vi "烟雾监测界面.vi"() -> ()   [LabVIEW 2016, in "环境动力监测库.lvlib"]
panel:
  out "x+1":u32
  in  "解除告警":bool
  out "告警内容":string
  out "X5-烟雾检测_YW":bool caption="状态"
  # "烟雾监测"
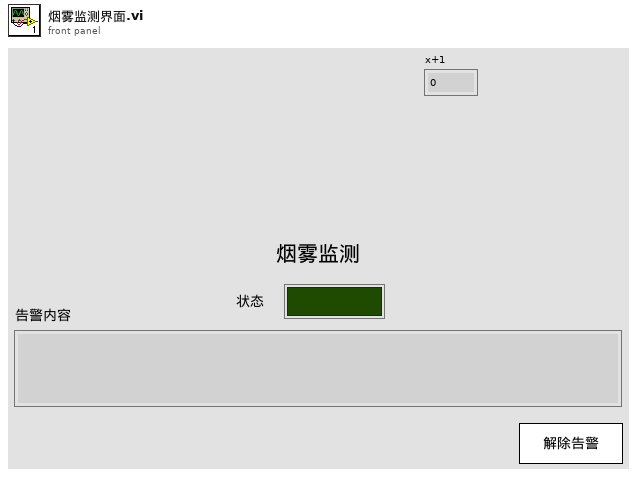
[diagram p1: front panel]
types:
  T1 = cluster{"漏水监测配置":cluster{"监测项描述:输出":string, "端口:":enum16{"AI0", "AI1", "AI2", "AI3", "AI4", "DI0", "DI1", "DI2", "DI3", "DI4", "DO0", "DO1", "DO2", "DO3", "DO4", "X0", "X1", "X2", "X3", "X4", "X5", "X6", "X7", "X8", "X9", "X10", "X11", "X12", "X13", "X14", "X15", "X16", "X17", "X18", "X19", "X20", "X21", "X22", "X23"}, "告警参数:":enum32{"禁用告警", "闭合告警", "断开告警"}, "传感器型号:":enum16{"PLC", "ZLAN", "ART"}, "声光告警启用":bool}, "门禁开关监测配置":cluster{"监测项描述:输出":string, "端口:":enum16{"AI0", "AI1", "AI2", "AI3", "AI4", "DI0", "DI1", "DI2", "DI3", "DI4", "DO0", "DO1", "DO2", "DO3", "DO4", "X0", "X1", "X2", "X3", "X4", "X5", "X6", "X7", "X8", "X9", "X10", "X11", "X12", "X13", "X14", "X15", "X16", "X17", "X18", "X19", "X20", "X21", "X22", "X23"}, "告警参数:":enum32{"禁用告警", "闭合告警", "断开告警"}, "传感器型号:":enum16{"PLC", "ZLAN", "ART"}, "声光告警启用":bool}, "门禁开关监测配置2":cluster{"监测项描述:输出":string, "端口:":enum16{"AI0", "AI1", "AI2", "AI3", "AI4", "DI0", "DI1", "DI2", "DI3", "DI4", "DO0", "DO1", "DO2", "DO3", "DO4", "X0", "X1", "X2", "X3", "X4", "X5", "X6", "X7", "X8", "X9", "X10", "X11", "X12", "X13", "X14", "X15", "X16", "X17", "X18", "X19", "X20", "X21", "X22", "X23"}, "告警参数:":enum32{"禁用告警", "闭合告警", "断开告警"}, "传感器型号:":enum16{"PLC", "ZLAN", "ART"}, "声光告警启用":bool}, "温湿度监测配置":cluster{"监测项描述:输出":string, "端口:":enum16{"AI0", "AI1", "AI2", "AI3", "AI4", "DI0", "DI1", "DI2", "DI3", "DI4", "DO0", "DO1", "DO2", "DO3", "DO4", "X0", "X1", "X2", "X3", "X4", "X5", "X6", "X7", "X8", "X9", "X10", "X11", "X12", "X13", "X14", "X15", "X16", "X17", "X18", "X19", "X20", "X21", "X22", "X23"}, "告警参数:":enum32{"禁用告警", "闭合告警", "断开告警"}, "传感器型号:":enum16{"PLC", "ZLAN", "ART"}, "声光告警启用":bool}, "烟雾监测配置":cluster{"监测项描述:输出":string, "端口:":enum16{"AI0", "AI1", "AI2", "AI3", "AI4", "DI0", "DI1", "DI2", "DI3", "DI4", "DO0", "DO1", "DO2", "DO3", "DO4", "X0", "X1", "X2", "X3", "X4", "X5", "X6", "X7", "X8", "X9", "X10", "X11", "X12", "X13", "X14", "X15", "X16", "X17", "X18", "X19", "X20", "X21", "X22", "X23"}, "告警参数:":enum32{"禁用告警", "闭合告警", "断开告警"}, "传感器型号:":enum16{"PLC", "ZLAN", "ART"}, "声光告警启用":bool}, "冰箱监测配置":cluster{"监测项描述:输出":string, "端口:":enum16{"AI0", "AI1", "AI2", "AI3", "AI4", "DI0", "DI1", "DI2", "DI3", "DI4", "DO0", "DO1", "DO2", "DO3", "DO4", "X0", "X1", "X2", "X3", "X4", "X5", "X6", "X7", "X8", "X9", "X10", "X11", "X12", "X13", "X14", "X15", "X16", "X17", "X18", "X19", "X20", "X21", "X22", "X23"}, "告警参数:":enum32{"禁用告警", "闭合告警", "断开告警"}, "传感器型号:":enum16{"PLC", "ZLAN", "ART"}, "声光告警启用":bool}, "排气扇监测配置":cluster{"监测项描述:输出":string, "端口:":enum16{"AI0", "AI1", "AI2", "AI3", "AI4", "DI0", "DI1", "DI2", "DI3", "DI4", "DO0", "DO1", "DO2", "DO3", "DO4", "X0", "X1", "X2", "X3", "X4", "X5", "X6", "X7", "X8", "X9", "X10", "X11", "X12", "X13", "X14", "X15", "X16", "X17", "X18", "X19", "X20", "X21", "X22", "X23"}, "告警参数:":enum32{"禁用告警", "闭合告警", "断开告警"}, "传感器型号:":enum16{"PLC", "ZLAN", "ART"}, "声光告警启用":bool}, "红外入侵监测配置":cluster{"监测项描述:输出":string, "端口:":enum16{"AI0", "AI1", "AI2", "AI3", "AI4", "DI0", "DI1", "DI2", "DI3", "DI4", "DO0", "DO1", "DO2", "DO3", "DO4", "X0", "X1", "X2", "X3", "X4", "X5", "X6", "X7", "X8", "X9", "X10", "X11", "X12", "X13", "X14", "X15", "X16", "X17", "X18", "X19", "X20", "X21", "X22", "X23"}, "告警参数:":enum32{"禁用告警", "闭合告警", "断开告警"}, "传感器型号:":enum16{"PLC", "ZLAN", "ART"}, "声光告警启用":bool}, "振动监测配置":cluster{"监测项描述:输出":string, "端口:":enum16{"AI0", "AI1", "AI2", "AI3", "AI4", "DI0", "DI1", "DI2", "DI3", "DI4", "DO0", "DO1", "DO2", "DO3", "DO4", "X0", "X1", "X2", "X3", "X4", "X5", "X6", "X7", "X8", "X9", "X10", "X11", "X12", "X13", "X14", "X15", "X16", "X17", "X18", "X19", "X20", "X21", "X22", "X23"}, "告警参数:":enum32{"禁用告警", "闭合告警", "断开告警"}, "传感器型号:":enum16{"PLC", "ZLAN", "ART"}, "声光告警启用":bool}}
  T2 = cluster{"监测项描述:输出":string, "端口:":enum16{"AI0", "AI1", "AI2", "AI3", "AI4", "DI0", "DI1", "DI2", "DI3", "DI4", "DO0", "DO1", "DO2", "DO3", "DO4", "X0", "X1", "X2", "X3", "X4", "X5", "X6", "X7", "X8", "X9", "X10", "X11", "X12", "X13", "X14", "X15", "X16", "X17", "X18", "X19", "X20", "X21", "X22", "X23"}, "告警参数:":enum32{"禁用告警", "闭合告警", "断开告警"}, "传感器型号:":enum16{"PLC", "ZLAN", "ART"}, "声光告警启用":bool}
  T3 = enum16{"AI0", "AI1", "AI2", "AI3", "AI4", "DI0", "DI1", "DI2", "DI3", "DI4", "DO0", "DO1", "DO2", "DO3", "DO4", "X0", "X1", "X2", "X3", "X4", "X5", "X6", "X7", "X8", "X9", "X10", "X11", "X12", "X13", "X14", "X15", "X16", "X17", "X18", "X19", "X20", "X21", "X22", "X23"}
  T4 = cluster{"状态":cluster{"R0":i16, "R1":i16, "R2":i16, "R3":i16, "R4":i16, "R5":i16, "R6":i16, "R7":i16, "R8":i16, "R9":i16, "R10":i16, "R11":i16, "R12":i16, "R13":i16, "R14":i16, "R15":i16, "R16":i16, "R17":i16, "R18":i16, "R19":i16, "R20":i16, "R21":i16, "R22":i16, "R23":i16, "R24":i16, "R25":i16, "R26":i16, "R27":i16, "R28":i16, "R29":i16, "R30":i16, "R31":i16, "R32":i16, "R33":i16, "R34":i16, "R35":i16, "R36":i16, "R37":i16, "R38":i16, "R39":i16}, "输入状态":bool[], "输出状态":bool[], "参数设置":cluster{"R100":i16, "R101":i16, "R102":i16, "R103":i16, "R104":i16, "R105":i16, "R106":i16, "R107":i16, "R108":i16, "R109":i16, "R110":i16, "R111":i16, "R112":i16, "R113":i16, "R114":i16, "R115":i16, "R116":i16, "R117":i16, "R118":i16, "R119":i16, "R120":i16, "R121":i16, "R122":i16, "R123":i16}, "转换值":cluster{"AD0":sgl, "AD1":sgl, "AD2":sgl, "AD3":sgl, "AD4":sgl, "AD5":sgl}}
  T5 = cluster{"状态":cluster{"R0":i16, "R1":i16, "R2":i16, "R3":i16, "R4":i16, "R5":i16, "R6":i16, "R7":i16, "R8":i16, "R9":i16, "R10":i16, "R11":i16, "R12":i16, "R13":i16, "R14":i16, "R15":i16, "R16":i16, "R17":i16, "R18":i16, "R19":i16, "R20":i16, "R21":i16, "R22":i16, "R23":i16, "R24":i16, "R25":i16, "R26":i16, "R27":i16, "R28":i16, "R29":i16, "R30":i16, "R31":i16, "R32":i16, "R33":i16, "R34":i16, "R35":i16, "R36":i16, "R37":i16, "R38":i16, "R39":i16, "R40":i16, "R41":i16, "R42":i16, "R43":i16, "R44":i16, "R45":i16, "R46":i16, "R47":i16, "R48":i16, "R49":i16, "R50":i16, "R51":i16, "R52":i16, "R53":i16, "R54":i16, "R55":i16, "R56":i16, "R57":i16, "R58":i16, "R59":i16, "R60":i16, "R61":i16, "R62":i16, "R63":i16, "R64":i16, "R65":i16, "R66":i16, "R67":i16, "R68":i16, "R69":i16}, "输入状态":bool[], "输出状态":bool[], "报警簇":bool[], "参数设置":cluster{"R100":i16, "R101":i16, "R102":i16, "R103":i16, "R104":i16, "R105":i16, "R106":i16, "R107":i16, "R108":i16, "R109":i16, "R110":i16, "R111":i16, "R112":i16, "R113":i16, "R114":i16, "R115":i16, "R116":i16, "R117":i16, "R118":i16, "R119":i16, "R120":i16, "R121":i16, "R122":i16, "R123":i16, "R124":i16}, "转换值":cluster{"AD0":sgl, "AD1":sgl, "AD2":sgl, "AD3":sgl, "AD4":sgl, "AD5":sgl}, "看门狗启用":bool, "氨氮模块名称":string, "总磷模块名称":string, "采配水模块类型":enum16{"V1", "V2", "V3", "V4", "室内V1", "室内V2"}}
  T6 = cluster{"环境变量":cluster{"蓄电池电压":dbl, "室温":dbl, "湿度":dbl, "水浸报警":bool, "烟雾报警":bool, "门禁1状态":bool, "门禁2状态":bool}, "ZLAN 6842 MB session":refnum<class "MB_Master.lvclass">, "DI":bool[], "DO":bool[]}
  T7 = cluster{"漏水监测输出":cluster{"漏水监测告警":bool, "告警内容":string}, "门禁监测输出":cluster{"门禁监测告警":bool, "告警内容":string}, "门禁监测输出2":cluster{"门禁监测告警":bool, "告警内容":string}, "温湿度监测输出":cluster{"温湿度监测告警":bool, "告警内容":string}, "烟雾监测输出":cluster{"烟雾监测告警":bool, "告警内容":string}, "空调监测输出":cluster{"空调监测告警":bool, "告警内容":string}, "自动重合闸输出":cluster{"自动重合闸告警":bool, "告警内容":string}, "红外入侵输出":cluster{"红外入侵告警":bool, "告警内容":string}, "振动输出":cluster{"振动告警":bool, "告警内容":string}, "UPS输出":cluster{"UPS告警":bool, "告警内容":string}, "蓄电池输出":cluster{"蓄电池告警":bool, "告警内容":string}, "蓄电池输出2":cluster{"蓄电池告警":bool, "告警内容":string}, "GPS输出":cluster{"定位告警":bool, "告警内容":string}, "北斗输出":cluster{"定位告警":bool, "告警内容":string}, "气象输出":cluster{"气象告警":bool, "告警内容":string}}
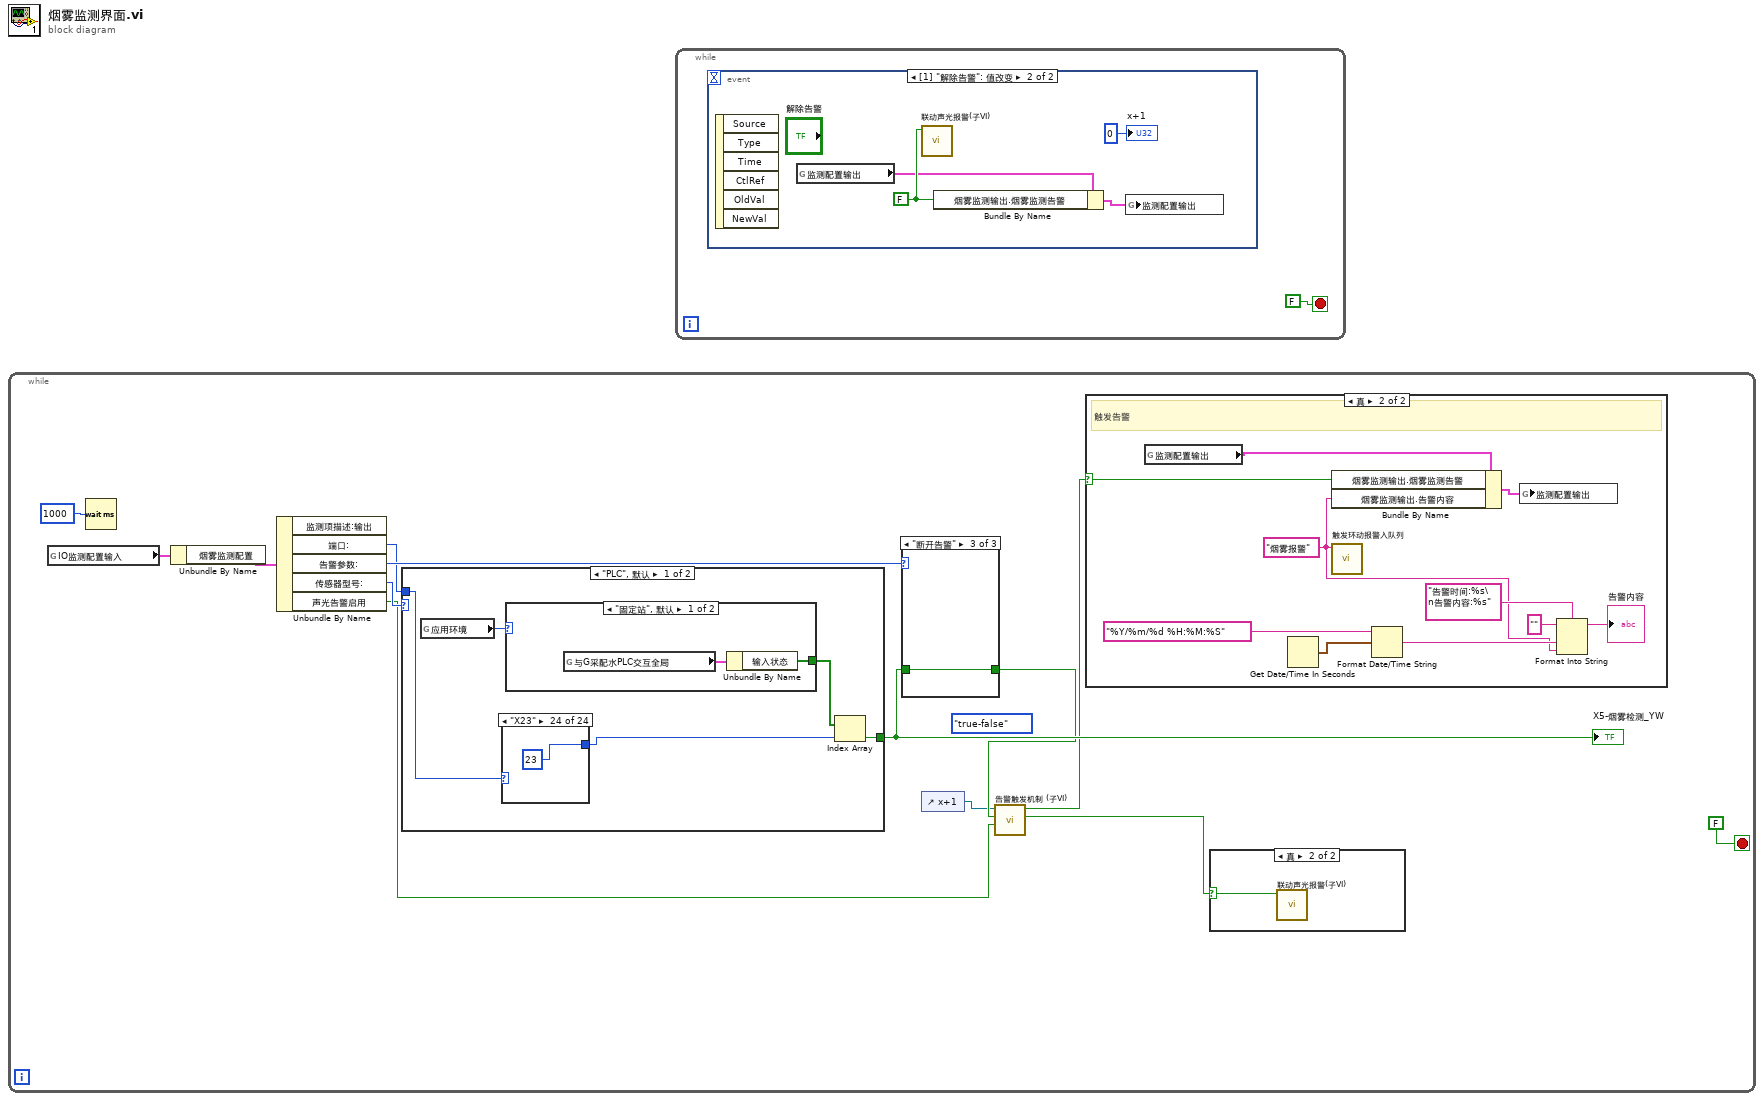
[diagram p0: block diagram]
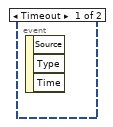
[diagram p2: hidden frame]
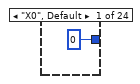
[diagram p4: hidden frame]
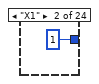
[diagram p5: hidden frame]
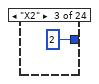
[diagram p6: hidden frame]
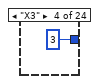
[diagram p7: hidden frame]
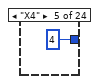
[diagram p8: hidden frame]
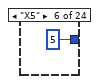
[diagram p9: hidden frame]
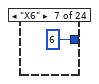
[diagram p10: hidden frame]
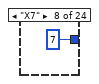
[diagram p11: hidden frame]
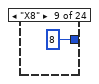
[diagram p12: hidden frame]
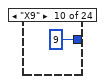
[diagram p13: hidden frame]
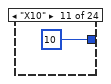
[diagram p14: hidden frame]
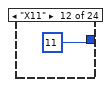
[diagram p15: hidden frame]
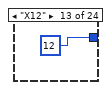
[diagram p16: hidden frame]
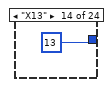
[diagram p17: hidden frame]
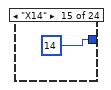
[diagram p18: hidden frame]
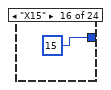
[diagram p19: hidden frame]
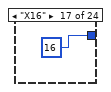
[diagram p20: hidden frame]
diagram:
  n1 = while {
    stop <- FALSE stop-if-true
    (unwired) enum16{"either", "false-true", "true-false"}."true-false" ("direction")
    n2 = global read "断电保存全局变量.vi" "IO监测配置输入"() -> (w9:T1)
    n3 = Wait (ms)(milliseconds to wait=u32 1000 ("等待时间（毫秒）")) -> ()  [unwired: 1 out]
    n4 = Unbundle By Name(w9) -> ("烟雾监测配置"=w13:T2)
    n5 = Unbundle By Name(w13) -> ("端口:"=w7:T3, "告警参数:"=w12:enum32{"禁用告警", "闭合告警", "断开告警"}, "传感器型号:"=w8:enum16{"PLC", "ZLAN", "ART"}, "声光告警启用"=w3:bool)  [unwired: 1 out]
    n6 = case shown="\"PLC\", 默认" w8 {
      tunnel: w7 -> [w16 w52]
      tunnel: [w19 w50] -> w6
      frame "PLC", Default {
        n7 = global read "外部交互全局变量.vi" "应用环境"() -> (w17:enum16{"固定站", "微站", "浮标", "浮船"})
        n8 = case shown="\"X23\"" w16 {
          tunnel: [0 ("索引") 1 ("索引") 2 ("索引") 3 ("索引") 4 ("索引") 5 ("索引") 6 ("索引") 7 ("索引") 8 ("索引") 9 ("索引") 10 ("索引") 11 ("索引") 12 ("索引") 13 ("索引") 14 ("索引") 15 ("索引") 16 ("索引") 17 ("索引") 18 ("索引") 19 ("索引") 20 ("索引") 21 ("索引") 22 ("索引") 23 ("索引")] -> w15
          frame "X0", Default {
          }
          frame "X1" {
          }
          frame "X2" {
          }
          frame "X3" {
          }
          frame "X4" {
          }
          frame "X5" {
          }
          frame "X6" {
          }
          frame "X7" {
          }
          frame "X8" {
          }
          frame "X9" {
          }
          frame "X10" {
          }
          frame "X11" {
          }
          frame "X12" {
          }
          frame "X13" {
          }
          frame "X14" {
          }
          frame "X15" {
          }
          frame "X16" {
          }
          frame "X17" {
          }
          frame "X18" {
          }
          frame "X19" {
          }
          frame "X20" {
          }
          frame "X21" {
          }
          frame "X22" {
          }
          frame "X23" {
          }
        }
        n9 = case shown="\"固定站\", 默认" w17 {
          tunnel: [w44 w46] -> w18
          frame "固定站", Default {
            n10 = global read "外部交互全局变量.vi" "与G采配水PLC交互全局"() -> (w45:T4)
            n11 = Unbundle By Name(w45) -> ("输入状态"=w44:bool[])
          }
          frame "微站" {
            n12 = global read "外部交互全局变量.vi" "与V采配水PLC交互全局"() -> (w47:T5)
            n13 = Unbundle By Name(w47) -> ("输入状态"=w46:bool[])
          }
        }
        n14 = Index Array(array=w18, index=w15) -> (element=w19:bool)
      }
      frame "ZLAN" {
        n15 = case shown="\"DI1\"" w52 {
          tunnel: [0 ("索引") 1 ("索引") 2 ("索引") 3 ("索引") 4 ("索引")] -> w51
          frame "DI0", Default {
          }
          frame "DI1" {
          }
          frame "DI2" {
          }
          frame "DI3" {
          }
          frame "DI4" {
          }
        }
        n16 = global read "外部交互全局变量.vi" "与ZLAN交互全局"() -> (w49:T6)
        n17 = Unbundle By Name(w49) -> ("DI"=w48:bool[])
        n18 = Index Array(array=w48, index=w51) -> (element=w50:bool)
      }
    }
    "X5-烟雾检测_YW" <- w6
    n19 = case shown="\"断开告警\"" w12 {
      tunnel: w6 -> [_ w70 w71]
      tunnel: [TRUE ("漏水监测输出") w69 w71] -> w2
      frame "禁用告警", Default {
      }
      frame "闭合告警" {
        n20 = Not(x=w70) -> (.not. x?=w69:bool)
      }
      frame "断开告警" {
      }
    }
    n21 = control-ref of="x+1"() -> (w1:refnum<vi>)
    n22 = call "告警触发机制 (子VI).vi"("声光告警启用"=w3, "状态输出"=w2, "Digital输入"=w1) -> ("声光告警"=w5:bool, "触发告警"=w4:bool)  [unwired: 7 in]
    n23 = case shown="真" w4 {
      selector: w4 -> [_ w67]
      frame False {
      }
      frame True {
        w61 = "烟雾报警" ("报警内容")
        # "触发告警"
        n24 = global read "内部交互全局变量.vi" "监测配置输出"() -> (w59:T7)
        n25 = Get Date/Time In Seconds() -> (seconds since 1Jan1904=w64:timestamp)
        n26 = Bundle By Name(cluster=w59, "烟雾监测输出.烟雾监测告警"=w67, "烟雾监测输出.告警内容"=w61) -> (w58:T7)
        n27 = call "触发环动报警入队列.vi"("报警内容"=w61) -> ()  [unwired: 11 in]
        n28 = Format Date/Time String(time format string (%c)="%Y/%m/%d %H:%M:%S" ("时间格式字符串(%c)"), seconds (now)=w64) -> (date/time string=w66:string)  [unwired: 1 in]
        n29 = global write "内部交互全局变量.vi" "监测配置输出"(w58) -> ()
        n30 = Format Into String(format string="告警时间:%s\n告警内容:%s" ("格式字符串"), initial string="" ("初始字符串"), w66, w61) -> (resulting string=→"告警内容":string)  [unwired: 1 in, 1 out]
      }
    }
    n31 = case shown="真" w5 {
      selector: w5 -> [_ w14]
      frame False {
      }
      frame True {
        n32 = call "联动声光报警(子VI).vi"("布尔"=w14) -> ()  [unwired: 11 in]
      }
    }
  }
  n33 = while {
    stop <- FALSE stop-if-true
    n34 = event shown="[1] \"解除告警\": 值改变" {
      selector: _ -> [_ _]
      dyn-events: _ -> [_ _]
      timeout: _ -> [_ _]
      event Timeout {
        n35 = event-data() -> ()  [unwired: 1 in, 3 out]
      }
      event "解除告警": Value Change {
        w76 = FALSE
        n36 = event-data() -> ()  [unwired: 1 in, 6 out]
        n37 = global read "内部交互全局变量.vi" "监测配置输出"() -> (w74:T7)
        n38 = call "联动声光报警(子VI).vi"("布尔"=w76) -> ()  [unwired: 11 in]
        n39 = Bundle By Name(cluster=w74, "烟雾监测输出.烟雾监测告警"=w76) -> (w73:T7)
        n40 = global write "内部交互全局变量.vi" "监测配置输出"(w73) -> ()
        "x+1" <- u32 0 ("x+1")
      }
    }
  }
